vi "ScanBox2Var_Asynchronous.vi"(0 "扫码项目":string[](array[string])=["SN："], 1 "Left(100)":i16=100, 2 "Top(100)":i16=100, 5 "扫码项长度":u32[](array[numeric]), 7 "扫码项文本头匹配":string[](array[string]), 9 "码不可重复":bool=TRUE, 11 "YTESTER测试数据":T1 caption="不要修改！", 12 "满足全部扫码后延迟触发测试（s）":dbl=-1.0, 13 "触发哪些DUTs自动测试？":string) -> ()   [LabVIEW 2017]
uses:
  YtCommon.lvlibp/yt`Step TestData.ctl
  YtCommon.lvlibp/yt`Step System Queue.ctl
  <vilib>/Utility/miscctls.llb/LVPointTypeDef.ctl
  <vilib>/Utility/miscctls.llb/LVRectTypeDef.ctl
  Step`s VIs Global.vi
  user32.dll
  YtCommon.lvlibp
panel:
  out "Timeuptips":string
  in  "OK Button":bool
  in  "聚焦":bool=TRUE
  in  "枪扫":bool=TRUE
  in  "置顶":bool=TRUE
  in  "SN10":string caption="erer"
  in  "SN9":string
  in  "SN8":string
  in  "SN7":string
  in  "SN6":string
  in  "SN5":string
  in  "SN4":string
  in  "SN3":string
  in  "SN2":string
  in  "SN1":string caption="SN："
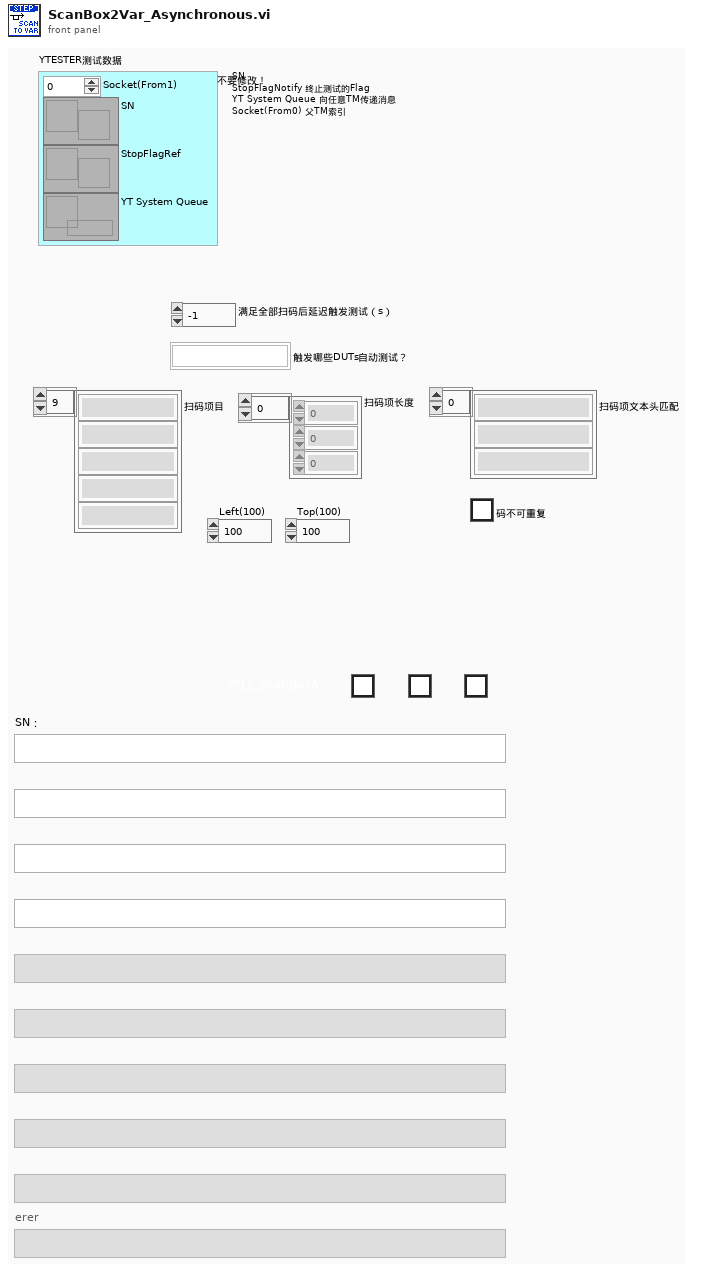
[diagram p1: front panel]
types:
  T1 = typedef "YtCommon.lvlibp/yt`Step TestData.ctl" = cluster{"Socket(From1)":i32, "SN":refnum<notifier>, "StopFlagRef":refnum<notifier>, "YT System Queue":refnum<queue>}
  T2 = typedef "LVPointTypeDef.ctl" = cluster{"Horizontal":i16, "Vertical":i16}
  T3 = enum32{"Invalid", "Standard", "Closed", "Hidden", "Minimized", "Maximized"}
  T4 = typedef "LVRectTypeDef.ctl" = cluster{"Left":i16, "Top":i16, "Right":i16, "Bottom":i16}
  T5 = typedef "YtCommon.lvlibp/yt`Step System Queue.ctl" = cluster{"Socket(From0)":i32, "Cmd":string, "Data":variant}
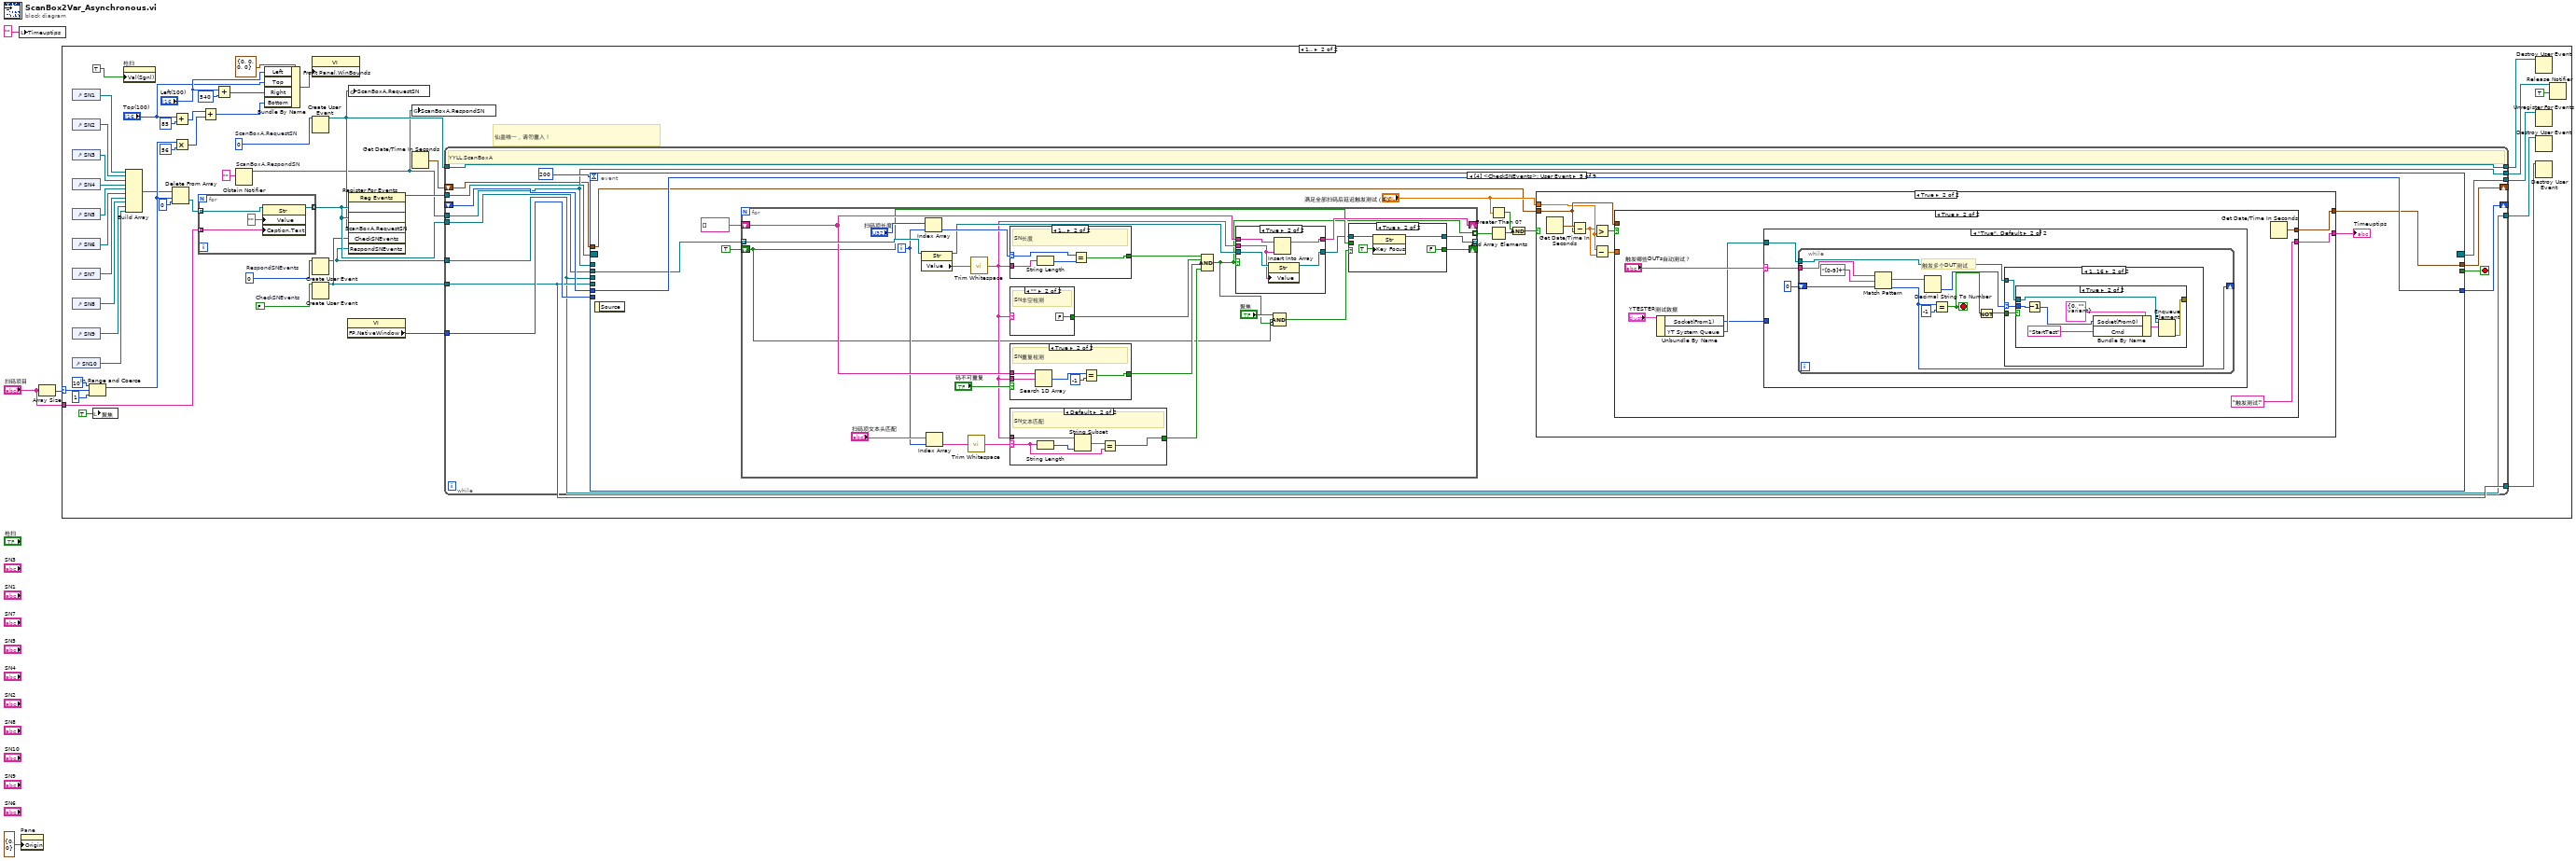
[diagram p0: block diagram]
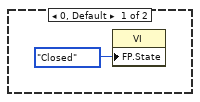
[diagram p2: hidden frame]
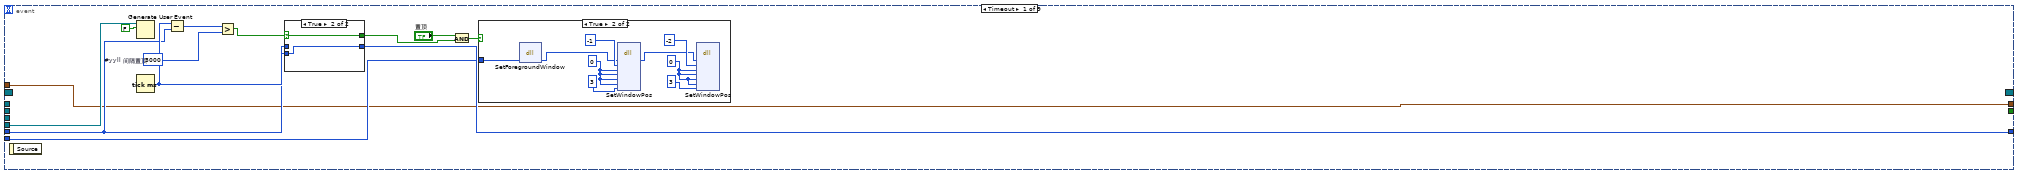
[diagram p3: hidden frame]
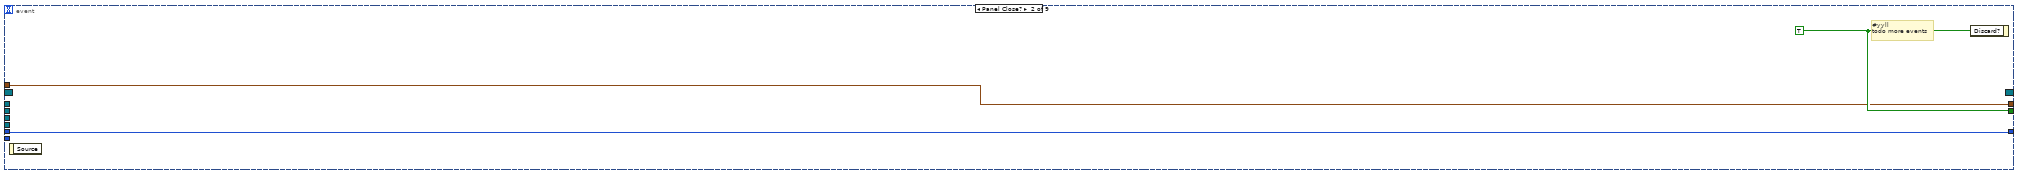
[diagram p6: hidden frame]
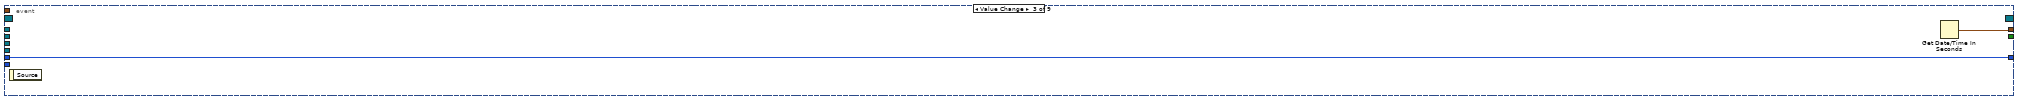
[diagram p7: hidden frame]
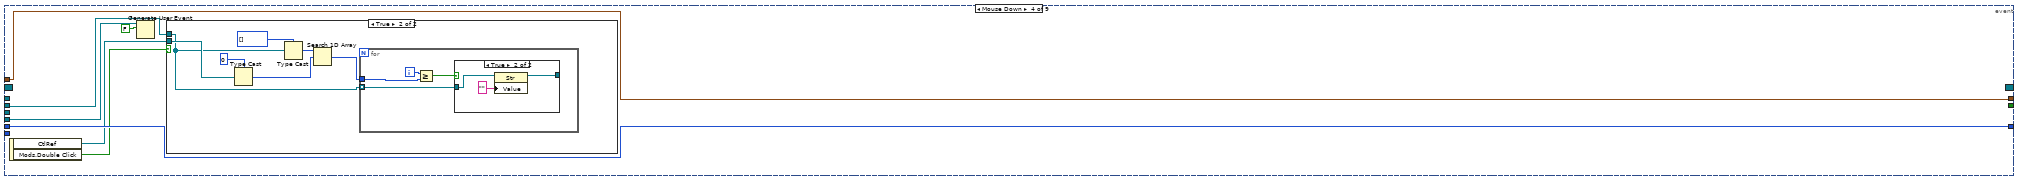
[diagram p8: hidden frame]
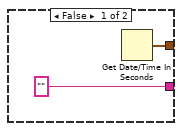
[diagram p11: hidden frame]
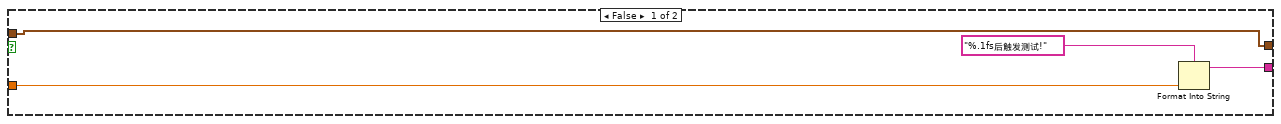
[diagram p12: hidden frame]
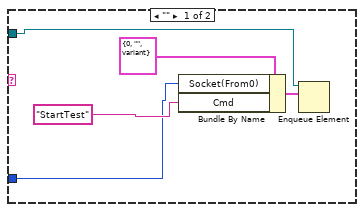
[diagram p13: hidden frame]
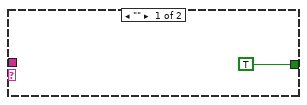
[diagram p17: hidden frame]
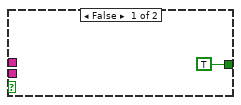
[diagram p18: hidden frame]
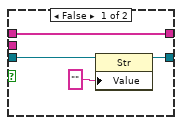
[diagram p19: hidden frame]
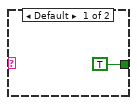
[diagram p20: hidden frame]
diagram:
  n1 = local write "Timeuptips"("" ("Timeuptips")) -> ()
  n2 = property on="Pane" class="Pane"("Origin"=T2 {"Horizontal"=0, "Vertical"=0}) -> ()  [unwired: 2 in, 2 out]
  n3 = Array Size(array="扫码项目") -> (size(s)=w3:i32)
  n4 = case shown="1.." w3 {
    selector: w3 -> [_ w27]
    tunnel: "扫码项目" -> [_ w23]
    frame 0, Default {
      n5 = property class="VI"("FP.State"=T3."Closed" ("前面板窗口:状态")) -> ()  [unwired: 2 in, 2 out]
    }
    frame 1.. {
      w9 = 0  # RespondSNEvents
      w13 = FALSE  # CheckSNEvents
      w20 = u32 0  # ScanBoxA.RequestSN
      # "仙蛊唯一，请勿重入！"
      n6 = control-ref of="SN1"() -> (w54:refnum<vi>)
      n7 = control-ref of="SN2"() -> (w52:refnum<vi>)
      n8 = control-ref of="SN3"() -> (w51:refnum<vi>)
      n9 = control-ref of="SN4"() -> (w50:refnum<vi>)
      n10 = control-ref of="SN5"() -> (w49:refnum<vi>)
      n11 = control-ref of="SN6"() -> (w48:refnum<vi>)
      n12 = control-ref of="SN7"() -> (w47:refnum<vi>)
      n13 = control-ref of="SN8"() -> (w46:refnum<vi>)
      n14 = control-ref of="SN9"() -> (w45:refnum<vi>)
      n15 = control-ref of="SN10"() -> (w44:refnum<vi>)
      n16 = In Range and Coerce(upper limit=10, x=w27, lower limit=1) -> (coerced(x)=w26:i32)  [unwired: 1 out]
      n17 = local write "聚焦"(TRUE ("聚焦")) -> ()
      n18 = property on="枪扫" class="Bool (strict)"("Val(Sgnl)"=TRUE ("Value (Signaling)")) -> ()  [unwired: 2 in, 2 out]
      n19 = Build Array(w54, w52, w51, w50, w49, w48, w47, w46, w45, w44) -> (w25:refnum<vi>[])
      n20 = Delete From Array(array=w25, length=w26, index=0) -> (deleted portion=w24:refnum<vi>[])  [unwired: 1 out]
      n21 = Add(x="Top(100)", y=i16 85) -> (x+y=w39:i16)
      n22 = Multiply(x=w26, y=56) -> (x*y=w38:i32)
      n23 = for {
        tunnel: w24 -> [w58] mode=indexing
        tunnel: [w57] -> w21 mode=indexing
        tunnel: w23 -> [w56] mode=indexing
        n24 = property on="Property Node" class="Str"(reference=w58, "Value"="", "Caption.Text"=w56) -> (reference out=w57:refnum<vi>)  [unwired: 1 in, 1 out]
      }
      n25 = Add(x=w39, y=w38) -> (x+y=w37:i32)
      n26 = Add(x="Left(100)", y=i16 540) -> (x+y=w42:i16)
      n27 = Obtain Notifier "ScanBoxA.RespondSN"(notification data type="") -> (notifier out=w14:refnum<notifier>)  [unwired: 3 in, 2 out]
      n28 = Bundle By Name(cluster=T4 {"Left"=0, "Top"=0, "Right"=0, "Bottom"=0} ("Front Panel Window:Window Bounds"), "Left"="Left(100)", "Top"="Top(100)", "Right"=w42, "Bottom"=w37) -> (w32:T4)
      n29 = property class="VI"("Front Panel.WinBounds"=w32) -> ()  [unwired: 2 in, 2 out]
      n30 = Create User Event(user event datatype=w20) -> (user event=w18:refnum<user-event>)  [unwired: 1 in, 1 out]
      n31 = Create User Event(user event datatype=w9) -> (user event=w8:refnum<user-event>)  [unwired: 1 in, 1 out]
      n32 = Create User Event(user event datatype=w13) -> (user event=w11:refnum<user-event>)  [unwired: 1 in, 1 out]
      n33 = property class="VI"() -> ("FP.NativeWindow"=w43:u64)  [unwired: 2 in, 2 out]
      n34 = global write "Step`s VIs Global.vi" "ScanBoxA.RequestSN"(w18) -> ()
      n35 = register-events(w21, w21, w18, w11, w8) -> (reference out=w53:refnum<event-registration>)  [unwired: 2 in, 1 out]
      n36 = global write "Step`s VIs Global.vi" "ScanBoxA.RespondSN"(w14) -> ()
      n37 = Get Date/Time In Seconds() -> (seconds since 1Jan1904=w6:timestamp)
      n38 = while {
        tunnel: w53 -> [w70]
        shift-right: [w69] -> _
        shift-left: _ -> [w68]
        tunnel: w43 -> [w67]
        tunnel: w21 -> [w66]
        tunnel: w18 -> [w65]
        tunnel: [w65] -> w19
        tunnel: w14 -> [w64]
        tunnel: [w64] -> w16
        tunnel: [w62] -> w12
        tunnel: w11 -> [w62]
        tunnel: [w63] -> w10
        tunnel: w8 -> [w61]
        tunnel: [w61] -> w7
        shift-right: [w60] -> _
        shift-left: w6 -> [w59]
        stop <- w71 stop-if-true
        # "YYLL.ScanBoxA"
        n39 = event shown="[4] <CheckSNEvents>: User Event" {
          selector: w70 -> [_ _ _ _ _ _ _ _ _]
          dyn-events: [_ _ _ _ _ _ _ _ _] -> w63
          timeout: 200 -> [_ _ _ _ _ _ _ _ _]
          tunnel: [_ w100 _ _ _ _ _ _ _] -> w71
          tunnel: [w79 w99 w102 w109 w136 w249 w263 w267 w271] -> w69
          tunnel: w68 -> [w78 w99 w102 w109 w136 w249 w263 w267 w271]
          tunnel: w67 -> [w76 _ _ _ _ _ _ _ _]
          tunnel: w66 -> [_ _ _ w106 w133 _ w259 _ w269]
          tunnel: w64 -> [_ _ _ _ _ _ w258 _ _]
          tunnel: w62 -> [w74 _ _ w104 _ w247 w252 _ _]
          tunnel: w61 -> [_ _ _ _ _ w246 _ _ _]
          tunnel: [w73 w98 w101 w103 w127 w243 w250 w264 w268] -> w60
          tunnel: w59 -> [w73 w98 _ w103 w126 w243 w250 w264 w268]
          event Timeout {
            w77 = u32 3000  # #yyll 间隔置顶
            n40 = event-data() -> ()  [unwired: 1 in, 1 out]
            n41 = Generate User Event(user event=w74, event data cluster=FALSE ("event data")) -> ()  [unwired: 2 in, 2 out]
            n42 = Tick Count (ms)() -> (millisecond timer value=w83:u32)
            n43 = Subtract(x=w83, y=w78) -> (x-y=w85:u32)
            n44 = Greater?(x=w85, y=w77) -> (0:w84:bool)
            n45 = case shown="True" w84 {
              selector: w84 -> [_ w96]
              tunnel: w83 -> [_ w97]
              tunnel: [w95 w97] -> w79
              tunnel: [_ w96] -> w82
              tunnel: w78 -> [w95 _]
              frame False {
              }
              frame True {
              }
            }
            n46 = And(x="置顶", y=w82) -> (x .and. y?=w80:bool)
            n47 = case shown="True" w80 {
              tunnel: w76 -> [_ w88]
              frame False {
              }
              frame True {
                w91 = 0 ("参数3")
                w92 = 0 ("参数3")
                n48 = dll-call lib="USER32.DLL" fn="SetForegroundWindow" label="闪烁获取焦点"("参数1"=w88) -> ("参数1"=w87:u32)  [unwired: 4 in, 2 out]
                n49 = dll-call lib="USER32.DLL" fn="SetWindowPos" label="置顶"("参数1"=w87, "参数2"=-1, "参数3"=w92, "参数4"=w92, "参数5"=w92, "参数6"=w92, "参数7"=3) -> ("参数1"=w86:u32)  [unwired: 10 in, 2 out]
                n50 = dll-call lib="USER32.DLL" fn="SetWindowPos" label="恢复"("参数1"=w86, "参数2"=-2, "参数3"=w91, "参数4"=w91, "参数5"=w91, "参数6"=w91, "参数7"=3 ("参数3")) -> ()  [unwired: 11 in, 2 out]
              }
            }
          }
          event Panel Close? {
            w100 = TRUE ("Discard?")
            # "#yyll\ntodo more events"
            n51 = event-data() -> ()  [unwired: 1 in, 1 out]
            n52 = event-data("Discard?"=w100) -> ()  [unwired: 1 in, 1 out]
          }
          event Value Change {
            n53 = event-data() -> ()  [unwired: 1 in, 1 out]
            n54 = Get Date/Time In Seconds() -> (seconds since 1Jan1904=w101:timestamp)
          }
          event Mouse Down {
            n55 = event-data() -> ("CtlRef"=w108:refnum<vi>, "Mods.Double Click"=w107:bool)  [unwired: 1 in]
            n56 = Generate User Event(user event=w104, event data cluster=FALSE ("event data")) -> ()  [unwired: 2 in, 2 out]
            n57 = case shown="True" w107 {
              tunnel: w108 -> [_ w116]
              tunnel: w106 -> [_ w115]
              frame False {
              }
              frame True {
                n58 = Type Cast(type=0 ("Numeric"), x=w116) -> (*(type *) &x=w113:i32)
                n59 = Type Cast(type=i32[] [], x=w115) -> (*(type *) &x=w112:i32[])
                n60 = Search 1D Array(1D array=w112, element=w113) -> (index of element=w114:i32)  [unwired: 1 in]
                n61 = for {
                  tunnel: w115 -> [w120] mode=indexing
                  tunnel: w114 -> [w117]
                  i -> [w119]
                  n62 = Greater Or Equal?(x=w119, y=w117) -> (x >= y?=w118:bool)
                  n63 = case shown="True" w118 {
                    tunnel: w120 -> [w121 w123]
                    tunnel: [w121 w122] -> _
                    frame False {
                    }
                    frame True {
                      n64 = property on="Property Node" class="Str"(reference=w123, "Value"="") -> (reference out=w122:refnum<vi>)  [unwired: 1 in, 1 out]
                    }
                  }
                }
              }
            }
          }
          event User Event {
            n65 = event-data() -> ()  [unwired: 1 in, 1 out]
            n66 = for {
              tunnel: w133 -> [w207] mode=indexing
              shift-right: [w201] -> _
              shift-left: string[] [] -> [w199]
              shift-right: [w189] -> _
              shift-left: TRUE -> [w188]
              tunnel: [w186] -> w132 mode=indexing
              tunnel: [w185] -> _ mode=indexing
              i -> [w194]
              n67 = property on="Property Node" class="Str"(reference=w207) -> (reference out=w202:refnum<vi>, "Value"=w206:string)  [unwired: 1 in, 1 out]
              n68 = Index Array(array="扫码项长度", index=w194) -> (element=w205:u32)
              n69 = Index Array(array="扫码项文本头匹配", index=w194) -> (element=w192:string)
              n70 = call <vilib>:"Trim Whitespace.vi"("string"=w192) -> ("trimmed string"=w193:string)  [unwired: 1 in]
              n71 = call <vilib>:"Trim Whitespace.vi"("string"=w206) -> ("trimmed string"=w196:string)  [unwired: 1 in]
              n72 = case shown="1.." w205 {
                selector: w205 -> [_ w241]
                tunnel: w196 -> [_ w242]
                tunnel: [TRUE w239] -> w204
                frame Default {
                }
                frame 1.. {
                  # "SN长度"
                  n73 = String Length(string=w242) -> (length=w240:i32)
                  n74 = Equal?(x=w241, y=w240) -> (x = y?=w239:bool)
                }
              }
              n75 = case shown="\"\"" w196 {
                tunnel: [TRUE FALSE] -> w203
                frame Default {
                }
                frame "" {
                  # "SN非空检测"
                }
              }
              n76 = case shown="True" "码不可重复" {
                tunnel: w196 -> [_ w222]
                tunnel: w199 -> [_ w223]
                tunnel: [TRUE w224] -> w198
                frame False {
                }
                frame True {
                  # "SN重复检测"
                  n77 = Search 1D Array(1D array=w223, element=w222) -> (index of element=w226:i32)  [unwired: 1 in]
                  n78 = Equal?(x=w226, y=-1) -> (x = y?=w224:bool)
                }
              }
              n79 = case shown="Default" w193 {
                selector: w193 -> [_ w219]
                tunnel: [TRUE w218] -> w197
                tunnel: w196 -> [_ w220]
                frame "" {
                }
                frame Default {
                  # "SN文本匹配"
                  n80 = String Length(string=w219) -> (length=w217:i32)
                  n81 = String Subset(string=w220, length (rest)=w217) -> (substring=w216:string)  [unwired: 1 in]
                  n82 = Equal?(x=w216, y=w219) -> (x = y?=w218:bool)
                }
              }
              n83 = Compound Arithmetic op=AND(w204, w203, w198, w197) -> (w186:bool)
              n84 = case shown="True" w186 {
                tunnel: w202 -> [w230 w235]
                tunnel: w196 -> [_ w231]
                tunnel: w199 -> [w229 w234]
                tunnel: [w229 w233] -> w201
                tunnel: [w228 w232] -> w187
                frame False {
                  n85 = property on="Property Node" class="Str"(reference=w230, "Value"="") -> (reference out=w228:refnum<vi>)  [unwired: 1 in, 1 out]
                }
                frame True {
                  n86 = property on="Property Node" class="Str"(reference=w235, "Value"=w231) -> (reference out=w232:refnum<vi>)  [unwired: 1 in, 1 out]
                  n87 = Insert Into Array(array=w234, new element=w231) -> (w233:string[])  [unwired: 1 in]
                }
              }
              n88 = Compound Arithmetic op=AND("聚焦", w188, invert w186) -> (w190:bool)
              n89 = case shown="True" w190 {
                tunnel: [w210 FALSE] -> w189
                tunnel: w188 -> [w210 _]
                tunnel: w187 -> [w209 w212]
                tunnel: [w209 w211] -> w185
                frame False {
                }
                frame True {
                  n90 = property on="Property Node" class="Str"(reference=w212, "Key Focus"=TRUE) -> (reference out=w211:refnum<vi>)  [unwired: 1 in, 1 out]
                }
              }
            }
            n91 = Greater Than 0?(x="满足全部扫码后延迟触发测试（s）") -> (x > 0?=w131:bool)
            n92 = And Array Elements(Boolean array=w132) -> (logical AND=w130:bool)
            n93 = And(x=w131, y=w130) -> (x .and. y?=w129:bool)
            n94 = case shown="True" w129 {
              tunnel: "满足全部扫码后延迟触发测试（s）" -> [_ w142]
              tunnel: [w138 w144] -> w127
              tunnel: w126 -> [_ w143]
              tunnel: ["" w139] -> w125
              frame False {
                n95 = Get Date/Time In Seconds() -> (seconds since 1Jan1904=w138:timestamp)
              }
              frame True {
                n96 = Get Date/Time In Seconds() -> (seconds since 1Jan1904=w146:timestamp)
                n97 = Subtract(x=w146, y=w143) -> (x-y=w141:dbl)
                n98 = Greater?(x=w141, y=w142) -> (0:w145:bool)
                n99 = Subtract(x=w142, y=w141) -> (x-y=w140:dbl)
                n100 = case shown="True" w145 {
                  tunnel: [w150 w156] -> w144
                  tunnel: w143 -> [w150 _]
                  tunnel: w140 -> [w148 _]
                  tunnel: [w147 "触发测试!" ("format string")] -> w139
                  frame False {
                    n101 = Format Into String(format string="%.1fs后触发测试!", w148) -> (resulting string=w147:string)  [unwired: 2 in, 1 out]
                  }
                  frame True {
                    n102 = Unbundle By Name("YTESTER测试数据") -> ("Socket(From1)"=w151:i32, "YT System Queue"=w152:refnum<queue>)
                    n103 = case shown="\"True\", Default" "触发哪些DUTs自动测试？" {
                      selector: "触发哪些DUTs自动测试？" -> [_ w162]
                      tunnel: w152 -> [w161 w163]
                      tunnel: w151 -> [w157 _]
                      frame "" {
                        n104 = Bundle By Name(cluster=T5 {"Socket(From0)"=0, "Cmd"="", "Data"=variant} ("element"), "Socket(From0)"=w157, "Cmd"="StartTest") -> (w159:T5)
                        n105 = Enqueue Element(queue=w161, element=w159) -> ()  [unwired: 2 in, 3 out]
                      }
                      frame "True", Default {
                        n106 = while {
                          shift-right: [w172] -> _
                          shift-left: 0 ("offset past match") -> [w173]
                          tunnel: w163 -> [w166]
                          tunnel: w162 -> [w165]
                          stop <- w169 stop-if-true
                          # "触发多个DUT测试"
                          n107 = Match Pattern(string=w165, regular expression="[0-9]+" ("format string"), offset (0)=w173) -> (match substring=w170:string, offset past match=w172:i32)  [unwired: 2 out]
                          n108 = Decimal String To Number(string=w170) -> (number=w167:i32)  [unwired: 2 in, 1 out]
                          n109 = Equal?(x=w172, y=-1) -> (x = y?=w169:bool)
                          n110 = Not(x=w169) -> (.not. x?=w168:bool)
                          n111 = case shown="1..16" w167 {
                            selector: w167 -> [_ w176]
                            tunnel: w168 -> [_ w175]
                            tunnel: w166 -> [_ w177]
                            frame 0, Default {
                            }
                            frame 1..16 {
                              n112 = case shown="True" w175 {
                                tunnel: w177 -> [_ w180]
                                tunnel: w176 -> [_ w179]
                                tunnel: [_ w178] -> _
                                frame False {
                                }
                                frame True {
                                n113 = Decrement(x=w179) -> (x-1=w184:i32)
                                n114 = Bundle By Name(cluster=T5 {"Socket(From0)"=0, "Cmd"="", "Data"=variant} ("element"), "Socket(From0)"=w184, "Cmd"="StartTest") -> (w183:T5)
                                n115 = Enqueue Element(queue=w180, element=w183) -> (error out=w178:errorcluster)  [unwired: 2 in, 2 out]
                                }
                              }
                            }
                          }
                        }
                      }
                    }
                    n116 = Get Date/Time In Seconds() -> (seconds since 1Jan1904=w156:timestamp)
                  }
                }
              }
            }
            "Timeuptips" <- w125
          }
          event User Event {
            n117 = event-data() -> ("ScanBoxA.RequestSN"=w244:u32)  [unwired: 1 in, 4 out]
            n118 = Generate User Event "#yyll 获取前要先计算一次---"(user event=w247, event data cluster=FALSE ("event data")) -> (error out=w245:errorcluster)  [unwired: 2 in, 1 out]
            n119 = Generate User Event "#yyll Respond"(user event=w246, event data cluster=w244, error in=w245) -> ()  [unwired: 1 in, 2 out]
          }
          event User Event {
            n120 = event-data() -> ("RespondSNEvents"=w257:i32)  [unwired: 1 in]
            n121 = Index Array(array=w259, index=w257) -> (element=w262:refnum<vi>)
            n122 = property on="Property Node" class="Str"(reference=w262) -> (reference out=w256:refnum<vi>, error out=w260:errorcluster, "Value"=w261:string)  [unwired: 1 in]
            n123 = Send Notification(notification=w261, notifier=w258, error in (no error)=w260) -> (error out=w254:errorcluster)  [unwired: 1 out]
            n124 = property on="Property Node" class="Str"(reference=w256, error in=w254, "Value"="") -> (error out=w253:errorcluster)  [unwired: 1 out]
            n125 = Generate User Event "#yyll 再计算一次---"(user event=w252, event data cluster=FALSE ("event data"), error in=w253) -> ()  [unwired: 1 in, 2 out]
          }
          event "OK Button": Mouse Down {
            n126 = event-data() -> ()  [unwired: 1 in, 1 out]
            n127 = property class="VI"("BDWin.Open"=TRUE ("Block Diagram Window:Open")) -> ()  [unwired: 2 in, 2 out]
            n128 = One Button Dialog(message="双击清除当前SN栏内容!\n聚焦：自动聚焦到最上面不符合项；\n枪扫：启用表示超时0.3s不输出会自动开始判断，适用于扫码枪；关闭适用于手动输入回车后；\n置顶：窗口周期0.3s到前端；") -> ()  [unwired: 1 in, 1 out]
          }
          event "枪扫": Value Change {
            n129 = event-data() -> ("NewVal"=w270:bool)  [unwired: 1 in]
            n130 = for {
              tunnel: w269 -> [w274] mode=indexing
              tunnel: w270 -> [w273]
              tunnel: [w272] -> _ mode=indexing
              n131 = property class="Str"(reference=w274, "UpdtWhileTyping"=w273) -> (reference out=w272:refnum<vi>)  [unwired: 1 in, 1 out]
            }
          }
        }
      }
      n132 = Destroy User Event(user event=w19) -> ()  [unwired: 1 in, 1 out]
      n133 = Unregister For Events(event registration refnum=w10) -> ()  [unwired: 1 in, 1 out]
      n134 = Destroy User Event(user event=w7) -> ()  [unwired: 1 in, 1 out]
      n135 = Destroy User Event(user event=w12) -> ()  [unwired: 1 in, 1 out]
      n136 = Release Notifier(notifier=w16, force destroy? (F)=TRUE) -> ()  [unwired: 1 in, 3 out]
    }
  }
